vi "Error Report.vi"(8 "error in (no error)":errorcluster, 11 "Instrument Handle In":i32) -> (0 "error out":errorcluster, 2 "Report":string, 3 "Instrument Handle Out":i32)   [LabVIEW 8.6, in "ZTScopeM.lvlib"]
doc: "Returns the most recent command string to cause an error."
uses:
  ZTScopeM.lvlib
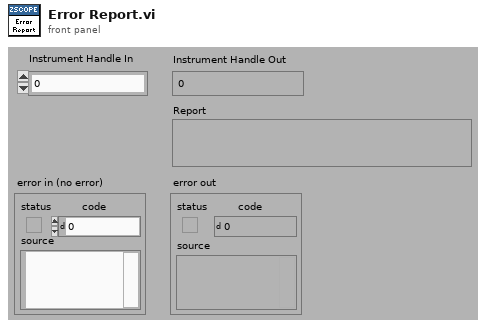
[diagram p1: front panel]
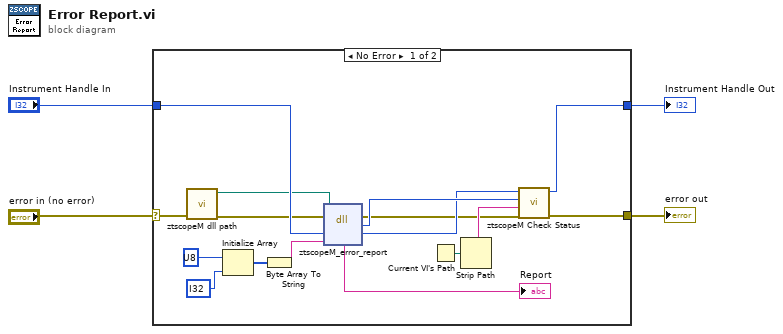
[diagram p0: block diagram]
diagram:
  n1 = case shown="No Error" "error in (no error)" {
    selector: "error in (no error)" -> [w8 w22]
    tunnel: [w17 w22] -> w3
    tunnel: "Instrument Handle In" -> [w19 w21]
    tunnel: [w18 w21] -> w1
    frame #0 {
      n2 = call "ztscopeM dll path.vi"("error in (no error)"=w8) -> ("error out"=w6:errorcluster, "<instrument>.dll path"=w7:path)  [unwired: 9 in]
      n3 = Initialize Array(u8 ? ("element"), i32 ? ("dimension size")) -> (w10:u8[])
      n4 = Byte Array To String(unsigned byte array=w10) -> (string=w9:string)
      n5 = dll-call lib="C:/Program Files (x86)/National Instruments/LabVIEW 2013/instr.lib/ztscopem/ztscopeM.dll" fn="ztscopeM_error_report"(path in=w7, error in=w6, "Instrument Handle"=w19, "Report"=w9) -> (error out=w5:errorcluster, "Status"=w15:i32, "Instrument Handle"=w14:i32, "Report"=→"Report":string)  [unwired: 1 in, 1 out]
      n6 = Current VI's Path() -> (path=w20:path)
      n7 = Strip Path(path=w20) -> (name=w16:string)  [unwired: 1 out]
      n8 = call "ztscopeM Check Status.vi"("error in"=w5, "name of VI"=w16, "status (return code)"=w15, "instrument handle in"=w14) -> ("error out"=w17:errorcluster, "instrument handle out"=w18:i32)  [unwired: 2 in]
    }
    frame #1 {
    }
  }
  "error out" <- w3
  "Instrument Handle Out" <- w1
